vi "Example_digital_out_control.vi"() -> ()   [LabVIEW 2022 SP3]
uses:
  usbtmc_scpi_labtool.lvlib
panel:
  in  "ID Query (True)":bool=TRUE
  in  "ID query string":string="PICO-PI,LABTOOL"
  in  "Exit on apply (F: Off)":bool
  in  "Apply Settings":bool
  in  "VISA resource name in":refnum<visa-resource-name>
  in  "Pin":u8 max=7 step=1
  in  "Enable Pin (F: Off)":bool
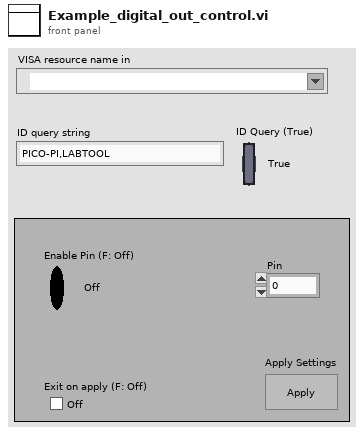
[diagram p1: front panel]
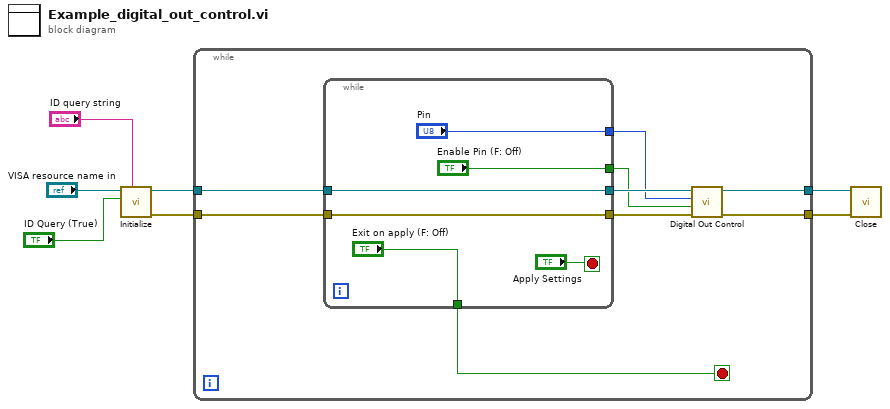
[diagram p0: block diagram]
diagram:
  n1 = call "Initialize.vi"("ID query string"="ID query string", "ID Query (True)"="ID Query (True)", "VISA resource name in"="VISA resource name in") -> ("error out"=w5:errorcluster, "VISA resource name out"=w7:refnum<visa-resource-name>)  [unwired: 7 in]
  n2 = while {
    tunnel: w7 -> [w14]
    tunnel: [w16] -> w6
    tunnel: w5 -> [w13]
    tunnel: [w15] -> w4
    stop <- w8 stop-if-true
    n3 = while {
      tunnel: w14 -> [w20]
      tunnel: w13 -> [w21]
      tunnel: [w21] -> w12
      tunnel: [w20] -> w11
      tunnel: ["Pin"] -> w10
      tunnel: ["Enable Pin (F: Off)"] -> w9
      tunnel: ["Exit on apply (F: Off)"] -> w8
      stop <- "Apply Settings" stop-if-true
    }
    n4 = call "Digital Out Control.vi"("VISA resource name"=w11, "Pin"=w10, "Enable Pin (F: Off)"=w9, "error in (no error)"=w12) -> ("VISA resource name out"=w16:refnum<visa-resource-name>, "error out"=w15:errorcluster)  [unwired: 5 in]
  }
  n5 = call "Close.vi"("error in (no error)"=w4, "VISA resource name"=w6) -> ()  [unwired: 10 in]
